vi "Send Pre-Addressed Unlock Publication.vi"(7 "Publisher ID":string, 8 "error in (no error)":errorcluster, 9 "Data to Publish":variant, 10 "Datum Name":string, 11 "Unlock Publication Msg":refnum<class "Unlock Publication Msg.lvclass">) -> (0 "error out":errorcluster)   [LabVIEW 2020, in "IMediator.lvlib" / "Unlock Publication Msg.lvclass"]
doc: "大多数想要发布数据的Actor或VI都会使用此send VI。调用此方法的Actor必须在发送之前收到预寻址的publish Msg。（对于Actor来说，这意味着它们是使用预寻址的发布消息启动的，或者是在中介激活后发送的。）"
uses:
  Unlock Publication Msg.lvclass
  Unlock Publication Msg.lvclass/Unlock Publication Msg.ctl
  composed-af-messages/Source/RoundTripMessage/RoundTripMessage.lvclass/RoundTripMessage.ctl
  <vilib>/ActorFramework/Message Enqueuer/Message Enqueuer.lvclass/Message Enqueuer.ctl
  <vilib>/ActorFramework/Message Enqueuer/Enqueue.vi
  composed-af-messages/Source/RoundTripMessage/RoundTripMessage.lvclass
  C:/Program Files/National Instruments/LabVIEW 2020/vi.lib/ActorFramework/Message/Message.lvclass
  <vilib>/ActorFramework/Message Priority Queue/Priority Enqueue.vi
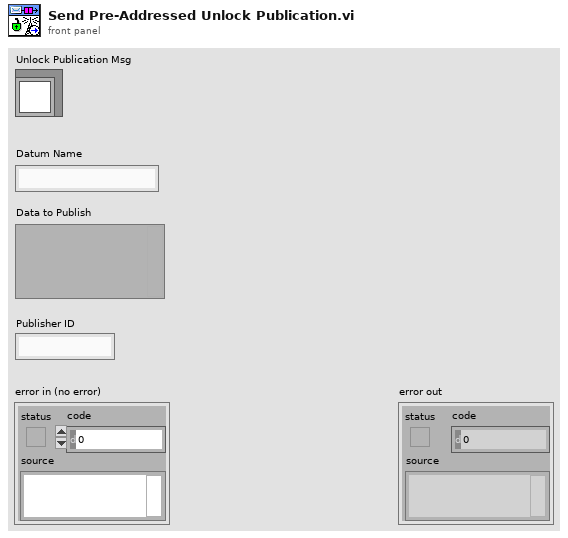
[diagram p1: front panel]
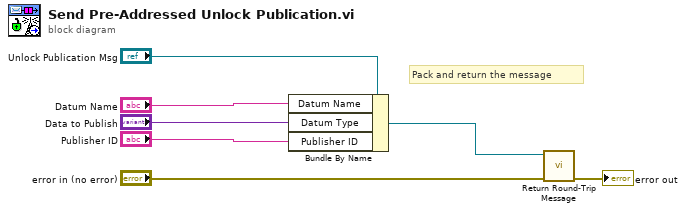
[diagram p0: block diagram]
diagram:
  # "Pack and return the message"
  n1 = Bundle By Name(cluster="Unlock Publication Msg", "Datum Name"="Datum Name", "Datum Type"="Data to Publish", "Publisher ID"="Publisher ID") -> (w3:refnum<class "Unlock Publication Msg.lvclass">)
  n2 = call "Return Round-Trip Message.vi"("error in (no error)"="error in (no error)", "RoundTripMessage In"=w3) -> ("error out"=→"error out":errorcluster)  [unwired: 9 in]
